vi "ReadCapBankShare.vi"(8 "error in (no error)":errorcluster, 11 "file path":path) -> (0 "error out":errorcluster, 1 "File size":i32, 2 "Text":string, 3 "Actual path":path)   [LabVIEW 2015]
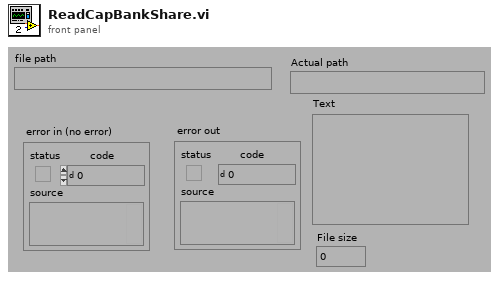
[diagram p1: front panel]
types:
  T1 = enum16{"read/write", "read-only", "write-only", "write-only (truncate)"}
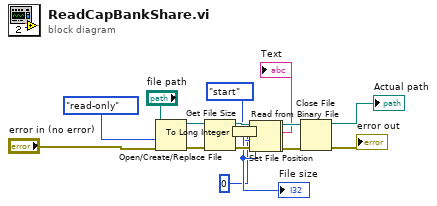
[diagram p0: block diagram]
diagram:
  n1 = Open/Create/Replace File(file path (use dialog)="file path", error in="error in (no error)", access (0:read/write)=T1."read-only" ("open mode (0)")) -> (refnum out=w15:refnum<file>, error out=w13:errorcluster)  [unwired: 4 out]
  n2 = Get File Size(file=w15, error in=w13) -> (refnum out=w14:refnum<file>, size (in bytes)=w3:i64, 0:w12:errorcluster)
  n3 = To Long Integer(number=w3) -> (32bit integer=w7:i32)
  "File size" <- w7
  n4 = Set File Position(offset (in bytes) (0)=0 ("pos offset (0)"), refnum=w14, from (0:start)=enum16{"start", "end", "current"}."start" ("pos mode (0:2)"), error in=w12) -> (refnum out=w2:refnum<file>, error out=w1:errorcluster)
  n5 = Read from Binary File(8:w1, 10:w7, 11:w2) -> (0:w11:errorcluster, 2:→"Text":string, 3:w9:refnum<file>)  [unwired: 4 out]
  n6 = Close File(refnum=w9, error in=w11) -> (path=→"Actual path":path, error out=→"error out":errorcluster)
